vi "Configure Digitize Input.vi"(6 "Buffer Name (\"\")":string, 7 "Count (0)":u32, 8 "error in (no error)":errorcluster, 10 "Block Number (1)":u32=1, 11 "VISA resource name":refnum<visa-resource-name>) -> (0 "error out":errorcluster, 3 "VISA resource name out":refnum<visa-resource-name>)   [LabVIEW 2023, in "Keithley DMM6500 DAQ6500 Series.lvlib"]
doc: "Defines a trigger block that makes a measurement using a digitize function."
uses:
  <instrlib>/Keithley DMM6500 DAQ6500 Series/Keithley DMM6500 DAQ6500 Series.lvlib
  <vilib>/Utility/error.llb/Trim Whitespace One-Sided.vi
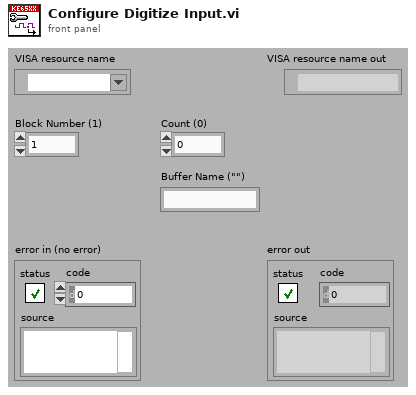
[diagram p1: front panel]
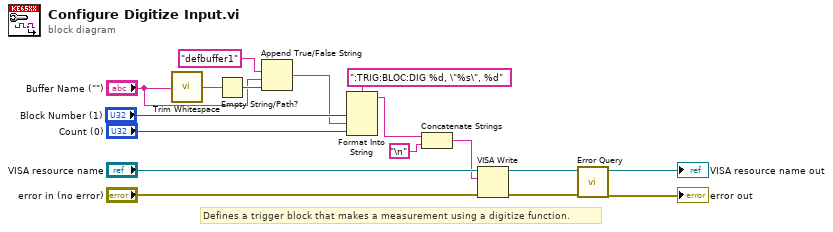
[diagram p0: block diagram]
diagram:
  # "Defines a trigger block that makes a measurement using a digitize function."
  n1 = call <vilib>:"Trim Whitespace.vi"("string"="Buffer Name (\"\")") -> ("trimmed string"=w5:string)  [unwired: 1 in]
  n2 = Empty String/Path?(string/path=w5) -> (empty?=w4:bool)
  n3 = Append True/False String(1:w4, 2:"Buffer Name (\"\")", 3:"defbuffer1" ("true string")) -> (0:w1:string)  [unwired: 1 in]
  n4 = Format Into String(format string=":TRIG:BLOC:DIG %d, \"%s\", %d", "Block Number (1)", w1, "Count (0)") -> (resulting string=w7:string)  [unwired: 2 in, 1 out]
  n5 = Concatenate Strings(w7, "\n") -> (w8:string)
  n6 = VISA Write(VISA resource name="VISA resource name", write buffer=w8, error in (no error)="error in (no error)") -> (VISA resource name out=w12:refnum<visa-resource-name>, error out=w11:errorcluster)  [unwired: 1 out]
  n7 = call <instrlib>:"Error Query.vi"("error in (no error)"=w11, "VISA resource name"=w12) -> ("error out"=→"error out":errorcluster, "VISA resource name out"=→"VISA resource name out":refnum<visa-resource-name>)  [unwired: 6 in, 2 out]
